vi "PH_PowerUnit_BaseClass.set i Attr and open Services.vi"(0 "i ref in":refnum<vi>, 5 "error in":errorcluster) -> (14 "i ref out":refnum<vi>, 16 "i Attribhutes":T1={"Constructor finished"=FALSE, "PU"={"In use"=FALSE, "Service ID in use"=-1, "GUI Ref"=refnum}, "Enabling"={"State"=0, "GUI Ref"=refnum}, "Timing"={"Last Shot"=0.0, "Time between Shots [Sec]"=30.0, "Waiting Time over?"=FALSE, "Service ID Waiting Time"=-1, "GUI Ref"=refnum, "Instance"={"Status"=0, "linked?"=FALSE, "GUI Ref"=refnum}}, "Sequencer"={"SM State"="N/A", "GUI Ref"=refnum, "linked"=FALSE}, "Subscribed Trendmssgs"=[], "PP PU"=enum."no Info", "Default Voltage (V)"=0.0, "GUI Refs"={"Delete Inst"=refnum, "State TO SM"=refnum, "State SM"=refnum, "Fire"=refnum}, "PSDB data"={"Shot Voltage [V]"=-1.0, "State TO SM"=enum.".", "Write 2 early"=FALSE}, "State TO SM"=enum."."} {"Subscribed Trendmssgs"."Shot Condition" items=["no info", "off/false/out", "on/true/in", "Failure", "Alarm", "Status 1", "Status 2", "Status 3"]; "Subscribed Trendmssgs"."Status" items=["no info", "off/false/out", "on/true/in", "Failure", "Alarm", "Status 1", "Status 2", "Status 3"]; "Timing"."Instance"."Status" items=["no info", "off/false/out", "on/true/in", "Failure", "Alarm", "Status 1", "Status 2", "Status 3"]; "Enabling"."State" items=["no info", "not disabled", "disabled"]}, 19 "error out":errorcluster)   [LabVIEW 2014, in "PH_PowerUnit_BaseClass.lvlib"]
doc: "In this VI the related instances which are not set in Read DB are set and written to own attributes as well as own DIM services are opened."
uses:
  PH_PowerUnit_BaseClass.lvlib
  PH_PowerUnit_BaseClass.i attribute.ctl
  PH_SystemInformation/PH_SystemInformationEnabling State.ctl
  PH_StatusHandler/PH_StatusHandler.Status.ctl
  PH_PP_Common/PH_PP_Common.PUs.ctl
  PH_PowerUnit_BaseClass.GUI Refs.ctl
  PH_PowerUnit_BaseClass.SM States.ctl
  PH_PowerUnit_BaseClass.PP PU Tags.ctl
  PH_Devices/PH_Beckhoff_PP_Control/PH_Beckhoff_PP_Control.PP Mercury Tags.ctl
  PH_Devices/PH_Beckhoff_PP_Control/PH_Beckhoff_PP_Control.PP Conductivity Tags.ctl
  PH_Devices/PH_Beckhoff-16BB/PH_Beckhoff-16BB.PA Chiller Tags.ctl
  PH_StatusHandler/PH_StatusHandler.lvlib
  PH_SystemInformation/PH_SystemInformation.lvlib
  CSlibraries-extern/DimLVEvent/LVDimInterface/LVDimInterface.lvlib
  PH_Common/PH_Common.lvlib
  CS_Core/CSSystem/CSSystemLib/CSSystemLib.lvlib
  PH_PP_Common/PH_PP_Common.lvlib
  PH_Devices/PH_Beckhoff-16BB/PH_Beckhoff-16BB.lvlib
  PH_Devices/PH_Beckhoff_PP_Control/PH_Beckhoff_PP_Control.lvlib
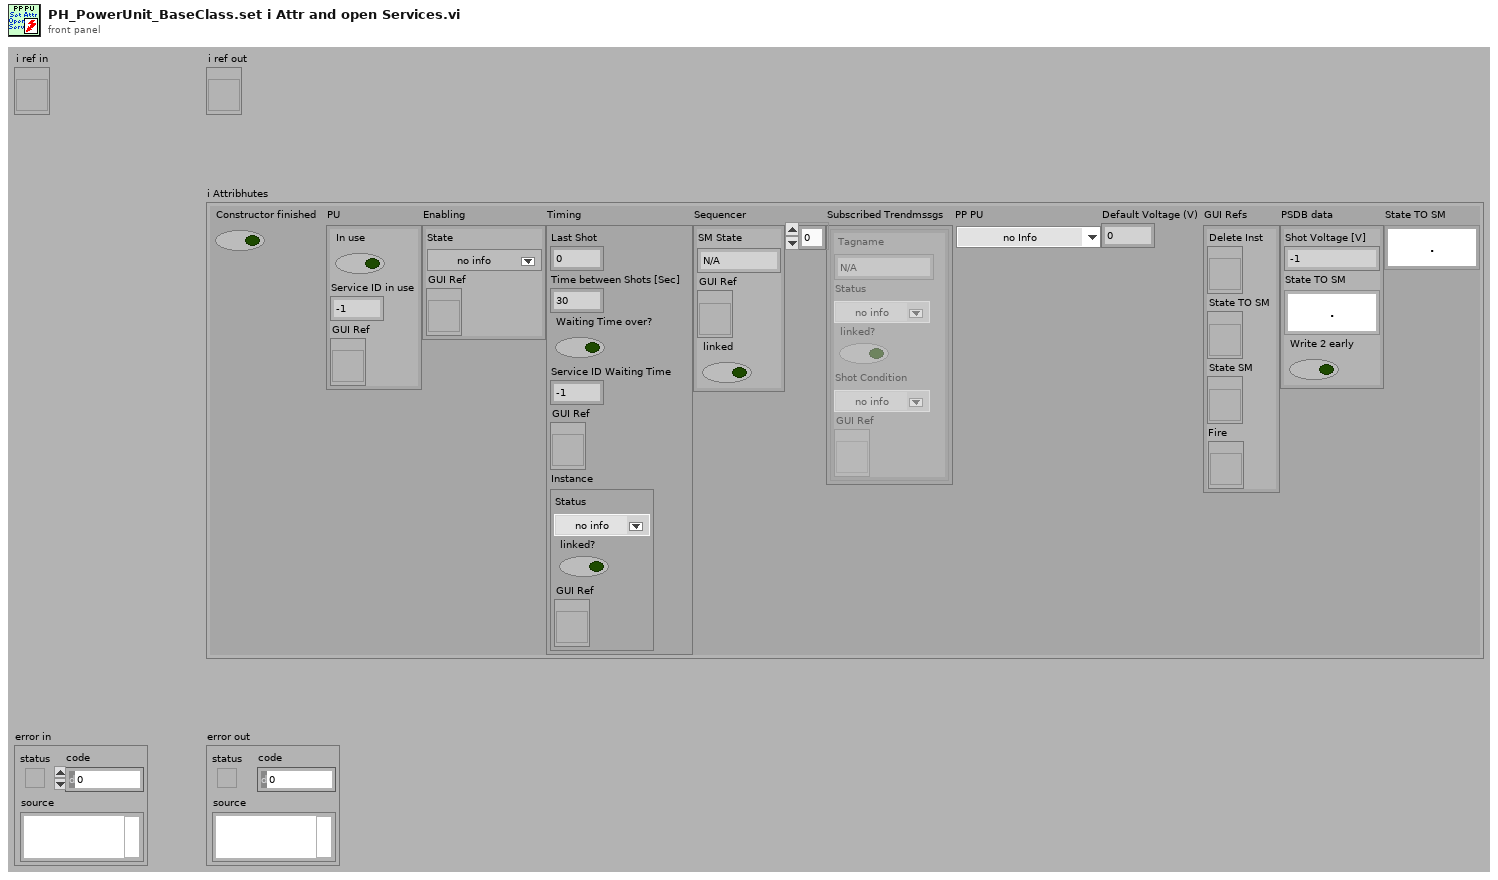
[diagram p1: front panel]
types:
  T1 = typedef "PH_PowerUnit_BaseClass.lvlib/PH_PowerUnit_BaseClass.i attribute.ctl" = cluster{"Constructor finished":bool, "PU":cluster{"In use":bool, "Service ID in use":i32, "GUI Ref":refnum<vi>}, "Enabling":cluster{"State":T2, "GUI Ref":refnum<vi>}, "Timing":cluster{"Last Shot":dbl, "Time between Shots [Sec]":dbl, "Waiting Time over?":bool, "Service ID Waiting Time":i32, "GUI Ref":refnum<vi>, "Instance":cluster{"Status":T3, "linked?":bool, "GUI Ref":refnum<vi>}}, "Sequencer":cluster{"SM State":string, "GUI Ref":refnum<vi>, "linked":bool}, "Subscribed Trendmssgs":cluster{"Tagname":string, "Status":T3, "linked?":bool, "Shot Condition":T3, "GUI Ref":refnum<vi>}[], "PP PU":T4, "Default Voltage (V)":dbl, "GUI Refs":T5, "PSDB data":cluster{"Shot Voltage [V]":dbl, "State TO SM":T6, "Write 2 early":bool}, "State TO SM":T6}
  T2 = typedef "PH_SystemInformation.lvlib/PH_SystemInformationEnabling State.ctl" = i32
  T3 = typedef "PH_StatusHandler.lvlib/PH_StatusHandler.Status.ctl" = i16
  T4 = typedef "PH_PP_Common.lvlib/PH_PP_Common.PUs.ctl" = enum16{"no Info", "PA-19mm-1", "PA-19mm-2", "PA-45mm-PILC", "PA-45mm-MAIN", "MA-PU-1", "MA-PU-2", "MA-PU-3", "MA-PU-4", "MA-PU-5", "MA-PU-6", "MA-FR", "MA-PILC", "PA-45mm-DP"}
  T5 = typedef "PH_PowerUnit_BaseClass.lvlib/PH_PowerUnit_BaseClass.GUI Refs.ctl" = cluster{"Delete Inst":refnum<vi>, "State TO SM":refnum<vi>, "State SM":refnum<vi>, "Fire":refnum<vi>}
  T6 = typedef "PH_PowerUnit_BaseClass.lvlib/PH_PowerUnit_BaseClass.SM States.ctl" = enum16{".", "Stand by", "Switch PU on", "Configure", "Set Default Voltage", "Set STANDBY", "Set READY", "Wait for Shot Cmd", "Open Dump Rods", "Open Ross Relais", "Close Ross Relais", "Switch PSU on", "Switch PSU off", "Charge", "Switch GD Channel on", "Close Dump Rods", "Rods-TO", "RR-TO", "PSU-TO", "Trigger-TO"}
  T7 = typedef "PH_PowerUnit_BaseClass.lvlib/PH_PowerUnit_BaseClass.PP PU Tags.ctl" = enum16{"Waiting-Time", "PU-in-Use"}
  T8 = typedef "PH_Beckhoff-16BB.lvlib/PH_Beckhoff-16BB.PA Chiller Tags.ctl" = enum16{"Flow-control", "High-temp", "Conductivity", "Niveau", "Status"}
  T9 = typedef "PH_Beckhoff_PP_Control.lvlib/PH_Beckhoff_PP_Control.PP Conductivity Tags.ctl" = enum16{"Device-on", "Conductivity-2-high", "Temperature-not-2-low", "Alarm", "Conductivity", "Status"}
  T10 = typedef "PH_Beckhoff_PP_Control.lvlib/PH_Beckhoff_PP_Control.PP Mercury Tags.ctl" = enum16{"Device-on", "Alarm", "on-since", "Concentration", "Status"}
  T11 = cluster{"Tagname":string, "Status":T3, "linked?":bool, "Shot Condition":T3, "GUI Ref":refnum<vi>}
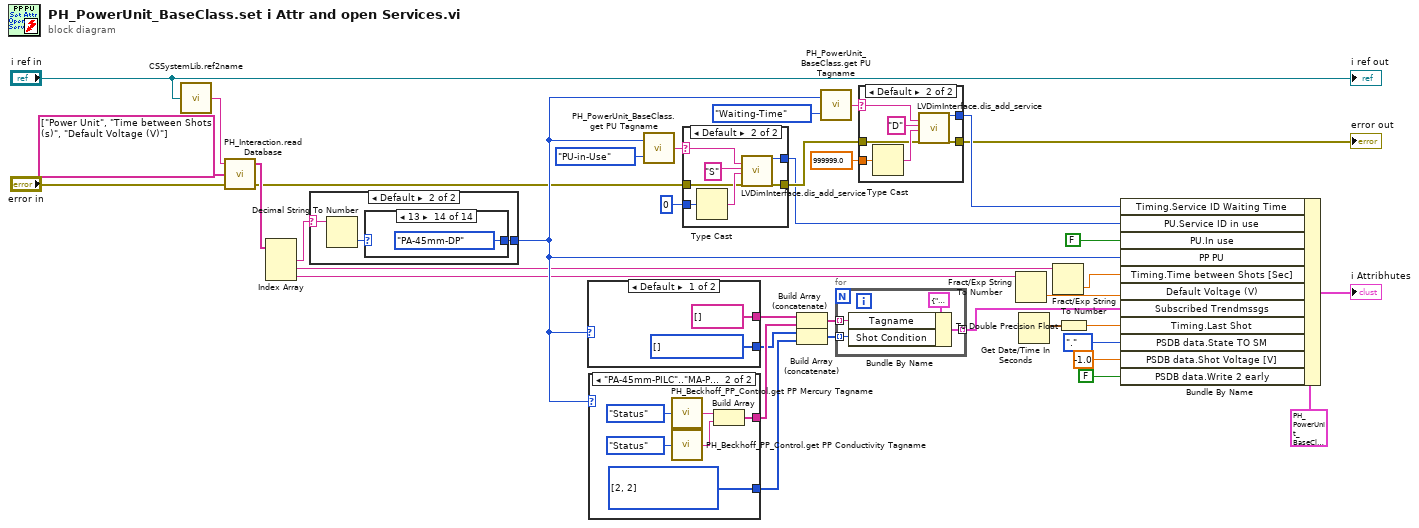
[diagram p0: block diagram]
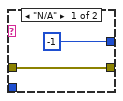
[diagram p2: hidden frame]
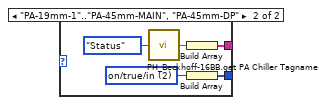
[diagram p3: hidden frame]
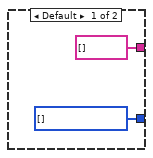
[diagram p4: hidden frame]
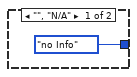
[diagram p5: hidden frame]
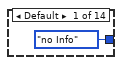
[diagram p6: hidden frame]
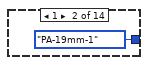
[diagram p7: hidden frame]
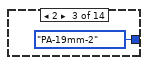
[diagram p8: hidden frame]
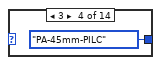
[diagram p9: hidden frame]
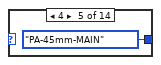
[diagram p10: hidden frame]
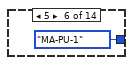
[diagram p11: hidden frame]
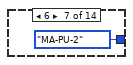
[diagram p12: hidden frame]
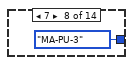
[diagram p13: hidden frame]
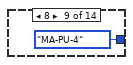
[diagram p14: hidden frame]
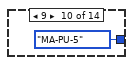
[diagram p15: hidden frame]
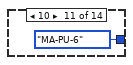
[diagram p16: hidden frame]
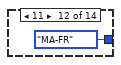
[diagram p17: hidden frame]
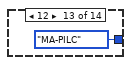
[diagram p18: hidden frame]
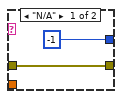
[diagram p19: hidden frame]
diagram:
  n1 = call "CSSystemLib.ref2name.vi"("obj refnum"="i ref in") -> ("name"=w30:string)
  n2 = call "PH_Interaction.read Database.vi"("error in (no error)"="error in", "Strings to search for"=string[] ["Power Unit", "Time between Shots (s)", "Default Voltage (V)"] ("Strings to search for in"), "DB Entry to read"=w30) -> ("error out"=w2:errorcluster, "Values"=w28:string[])  [unwired: 1 in]
  n3 = Index Array(array=w28) -> (element #1=w26:string, element #2=w11:string, element #3=w10:string)  [unwired: 3 in]
  n4 = case shown="Default" w26 {
    selector: w26 -> [_ w41]
    tunnel: [PH_PP_Common.PUs."no Info" ("PU") w39] -> w12
    frame "", "N/A" {
    }
    frame Default {
      n5 = Decimal String To Number(string=w41) -> (number=w40:i32)  [unwired: 2 in, 1 out]
      n6 = case shown="13" w40 {
        tunnel: [PH_PP_Common.PUs."no Info" ("PU") PH_PP_Common.PUs."PA-19mm-1" ("PU") PH_PP_Common.PUs."PA-19mm-2" ("PU") PH_PP_Common.PUs."PA-45mm-PILC" ("PU") PH_PP_Common.PUs."PA-45mm-MAIN" ("PU") PH_PP_Common.PUs."MA-PU-1" ("PU") PH_PP_Common.PUs."MA-PU-2" ("PU") PH_PP_Common.PUs."MA-PU-3" ("PU") PH_PP_Common.PUs."MA-PU-4" ("PU") PH_PP_Common.PUs."MA-PU-5" ("PU") PH_PP_Common.PUs."MA-PU-6" ("PU") PH_PP_Common.PUs."MA-FR" ("PU") PH_PP_Common.PUs."MA-PILC" ("PU") PH_PP_Common.PUs."PA-45mm-DP" ("PU")] -> w39
        frame Default {
        }
        frame 1 {
        }
        frame 2 {
        }
        frame 3 {
        }
        frame 4 {
        }
        frame 5 {
        }
        frame 6 {
        }
        frame 7 {
        }
        frame 8 {
        }
        frame 9 {
        }
        frame 10 {
        }
        frame 11 {
        }
        frame 12 {
        }
        frame 13 {
        }
      }
    }
  }
  n7 = case shown="Default" w12 {
    tunnel: [w56 w59] -> w18
    tunnel: [string[] [] w58] -> w17
    frame Default {
      w56 = T3[] [] items=["no info", "off/false/out", "on/true/in", "Failure", "Alarm", "Status 1", "Status 2", "Status 3"]
    }
    frame "PA-19mm-1".."PA-45mm-MAIN", "PA-45mm-DP" {
      w61 = T3 2 items=["no info", "off/false/out", "on/true/in", "Failure", "Alarm", "Status 1", "Status 2", "Status 3"] ("Shot Condition")
      n8 = call "PH_Beckhoff-16BB.get PA Chiller Tagname.vi"("PA Chiller Tag"=PH_Beckhoff-16BB.PA_Chiller_Tags."Status") -> ("PA Chiller Tagname"=w60:string)
      n9 = Build Array(w60) -> (w58:string[])
      n10 = Build Array(w61) -> (w59:T3[])
    }
  }
  n11 = case shown="\"PA-45mm-PILC\"..\"MA-PILC\"" w12 {
    tunnel: [string[] [] w66] -> w20
    tunnel: [w63 w65] -> w19
    frame Default {
      w63 = T3[] [] items=["no info", "off/false/out", "on/true/in", "Failure", "Alarm", "Status 1", "Status 2", "Status 3"]
    }
    frame "PA-45mm-PILC".."MA-PILC" {
      w65 = T3[] [2, 2] items=["no info", "off/false/out", "on/true/in", "Failure", "Alarm", "Status 1", "Status 2", "Status 3"]
      n12 = call "PH_Beckhoff_PP_Control.get PP Mercury Tagname.vi"("PP Mercury Tag"=PH_Beckhoff_PP_Control.PP_Mercury_Tags."Status") -> ("PP Mercury Tagname"=w67:string)
      n13 = call "PH_Beckhoff_PP_Control.get PP Conductivity Tagname.vi"("PP Conductivity Tag"=PH_Beckhoff_PP_Control.PP_Conductivity_Tags."Status") -> ("PP Conductivity Tagname"=w70:string)
      n14 = Build Array(w67, w70) -> (w66:string[])
    }
  }
  n15 = call "PH_PowerUnit_BaseClass.get PU Tagname.vi"("PU Tag"=PH_PowerUnit_BaseClass.PP_PU_Tags."PU-in-Use", "PU"=w12) -> ("PU Tagname"=w5:string)
  n16 = case shown="Default" w5 {
    selector: w5 -> [_ w75]
    tunnel: [-1 ("my_serviceID") w76] -> w4
    tunnel: [w71 w77] -> w22
    tunnel: w2 -> [w71 w74]
    tunnel: i16 0 ("Number") -> [_ w73]
    frame "N/A" {
    }
    frame Default {
      n17 = Type Cast(x=w73) -> (*(type *) &x=w79:string)  [unwired: 1 in]
      n18 = call "LVDimInterface.dis_add_service.vi"("serviceName"=w75, "typeDescriptor"="S", "data"=w79, "error in (no error)"=w74) -> ("my_serviceID"=w76:i32, "error out"=w77:errorcluster)  [unwired: 14 in]
    }
  }
  n19 = Build Array (concatenate)(w17, w20) -> (w16:string[])
  n20 = Build Array (concatenate)(w18, w19) -> (w15:T3[])
  n21 = call "PH_PowerUnit_BaseClass.get PU Tagname.vi"("PU Tag"=PH_PowerUnit_BaseClass.PP_PU_Tags."Waiting-Time", "PU"=w12) -> ("PU Tagname"=w24:string)
  n22 = for {
    tunnel: [w83] -> w35 mode=indexing
    tunnel: w16 -> [w81] mode=indexing
    tunnel: w15 -> [w80] mode=indexing
    n23 = Bundle By Name(cluster=T11 {"Tagname"="", "Status"=0, "linked?"=FALSE, "Shot Condition"=0, "GUI Ref"=refnum} ("Device"), "Tagname"=w81, "Shot Condition"=w80) -> (w83:T11)
  }
  n24 = case shown="Default" w24 {
    selector: w24 -> [_ w87]
    tunnel: [-1 ("my_serviceID") w89] -> w23
    tunnel: [w84 w90] -> w21
    tunnel: 999999.0 ("element") -> [_ w88]
    tunnel: w22 -> [w84 w86]
    frame "N/A" {
    }
    frame Default {
      n25 = Type Cast(x=w88) -> (*(type *) &x=w92:string)  [unwired: 1 in]
      n26 = call "LVDimInterface.dis_add_service.vi"("serviceName"=w87, "typeDescriptor"="D", "data"=w92, "error in (no error)"=w86) -> ("my_serviceID"=w89:i32, "error out"=w90:errorcluster)  [unwired: 14 in]
    }
  }
  "error out" <- w21
  n27 = Fract/Exp String To Number(string=w10) -> (number=w14:dbl)  [unwired: 3 in, 1 out]
  n28 = Get Date/Time In Seconds() -> (seconds since 1Jan1904=w36:timestamp)
  n29 = Fract/Exp String To Number(string=w11) -> (number=w27:dbl)  [unwired: 3 in, 1 out]
  n30 = To Double Precision Float(number=w36) -> (double precision float=w33:dbl)
  n31 = Bundle By Name(cluster=T1 {"Constructor finished"=FALSE, "PU"={"In use"=FALSE, "Service ID in use"=0, "GUI Ref"=refnum}, "Enabling"={"State"=0, "GUI Ref"=refnum}, "Timing"={"Last Shot"=0.0, "Time between Shots [Sec]"=0.0, "Waiting Time over?"=FALSE, "Service ID Waiting Time"=0, "GUI Ref"=refnum, "Instance"={"Status"=0, "linked?"=FALSE, "GUI Ref"=refnum}}, "Sequencer"={"SM State"="", "GUI Ref"=refnum, "linked"=FALSE}, "Subscribed Trendmssgs"=[], "PP PU"=enum."no Info", "Default Voltage (V)"=0.0, "GUI Refs"={"Delete Inst"=refnum, "State TO SM"=refnum, "State SM"=refnum, "Fire"=refnum}, "PSDB data"={"Shot Voltage [V]"=0.0, "State TO SM"=enum.".", "Write 2 early"=FALSE}, "State TO SM"=enum."."} ("i attribute"), "Timing.Service ID Waiting Time"=w23, "PU.Service ID in use"=w4, "PU.In use"=FALSE, "PP PU"=w12, "Timing.Time between Shots [Sec]"=w27, "Default Voltage (V)"=w14, "Subscribed Trendmssgs"=w35, "Timing.Last Shot"=w33, "PSDB data.State TO SM"=PH_PowerUnit_BaseClass.SM_States.".", "PSDB data.Shot Voltage [V]"=-1.0, "PSDB data.Write 2 early"=FALSE) -> (→"i Attribhutes":T1)
  "i ref out" <- "i ref in"
